vi "Get File Handle.vi"(8 "error in (no error)":errorcluster, 11 "Logger in":refnum<class "Logger.lvclass">) -> (0 "error out":errorcluster, 1 "Valid":bool, 2 "File handle":refnum<k34>, 3 "Logger out":refnum<class "Logger.lvclass">, 5 "Data File  Path":path)   [LabVIEW 2016, in "Logger.lvclass"]
uses:
  Logger.lvclass
  Logger.lvclass/Logger.ctl
  NHMFL_Core/Libraries/File/File Class/File.lvclass/File.ctl
  Read File.lvclass.vi
  NHMFL_Core/Libraries/File/File Class/Read tdms stream.vi
  NHMFL_Core/Libraries/File/File Class/Read Is open.vi
  NHMFL_Core/Libraries/File/File Class/Read Data File  Path.vi
  NHMFL_Core/Libraries/File/File Class/File.lvclass
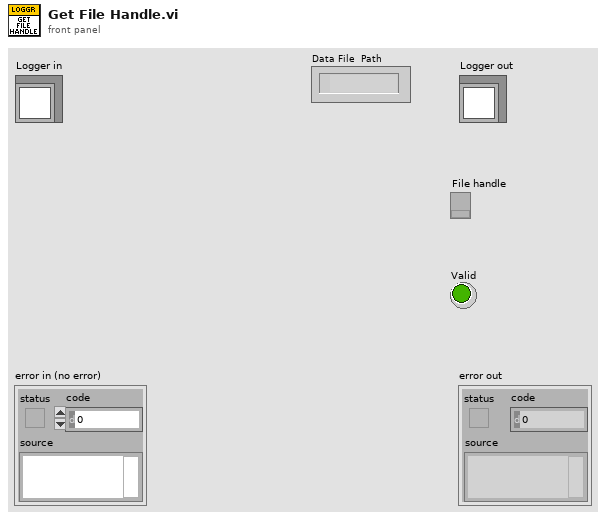
[diagram p1: front panel]
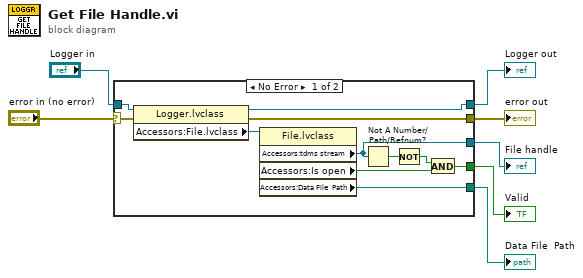
[diagram p0: block diagram]
diagram:
  n1 = case shown="No Error" "error in (no error)" {
    selector: "error in (no error)" -> [w18 w20]
    tunnel: [w17 w20] -> w6
    tunnel: [w15 w19] -> w4
    tunnel: "Logger in" -> [w16 w19]
    tunnel: [w13 _] -> w3
    tunnel: [w9 _] -> w2
    tunnel: [w8 _] -> w1
    frame No Error {
      n2 = property class="Logger.lvclass"(reference=w16, error in=w18) -> (reference out=w15:refnum<class "Logger.lvclass">, error out=w17:errorcluster, "Accessors:File.lvclass"=w14:refnum<class "File.lvclass">)
      n3 = property class="File.lvclass"(reference=w14) -> ("Accessors:tdms stream"=w13:refnum<k34>, "Accessors:Is open"=w10:bool, "Accessors:Data File  Path"=w8:path)  [unwired: 1 in, 2 out]
      n4 = Not A Number/Path/Refnum?(number/path/refnum=w13) -> (NaN/Path/Refnum?=w12:bool)
      n5 = Not(x=w12) -> (.not. x?=w11:bool)
      n6 = And(x=w11, y=w10) -> (x .and. y?=w9:bool)
    }
    frame Error {
    }
  }
  "error out" <- w6
  "Logger out" <- w4
  "File handle" <- w3
  "Valid" <- w2
  "Data File  Path" <- w1
